vi "jog motor.vi"(8 "error in (no error)":errorcluster, 10 "CCW? (T)":bool=TRUE, 11 "Stepper in":refnum<class "Stepper.lvclass">) -> (0 "error out":errorcluster, 3 "Stepper out":refnum<class "Stepper.lvclass">)   [LabVIEW 2025, in "Motor.lvlib" / "Stepper.lvclass"]
uses:
  Stepper.lvclass
  Stepper.lvclass/Stepper.ctl
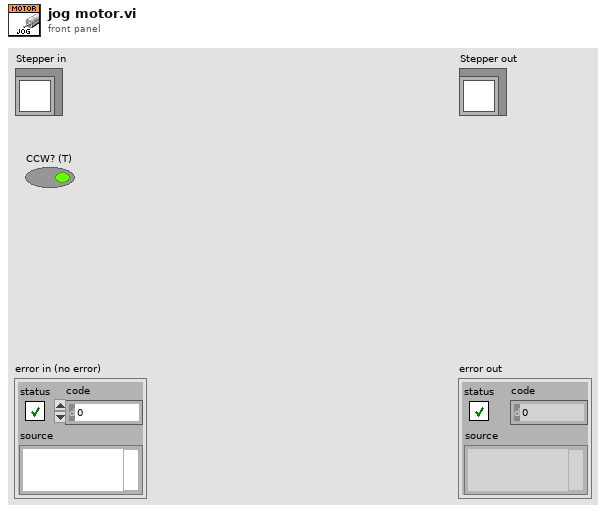
[diagram p1: front panel]
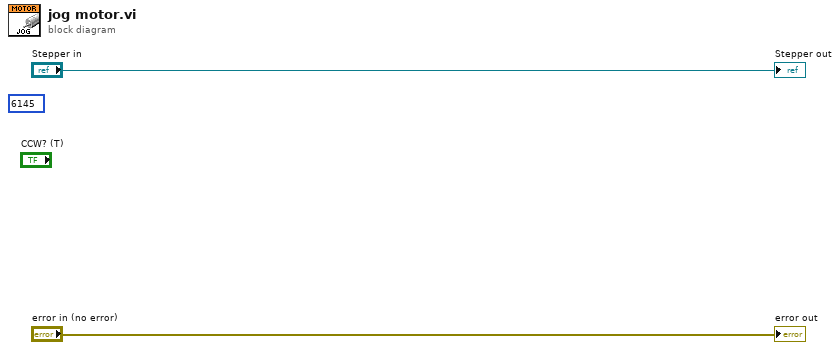
[diagram p0: block diagram]
diagram:
  (unwired) u16 6145 ("address")
  "error out" <- "error in (no error)"
  "Stepper out" <- "Stepper in"
